vi "Vision Global.vi"() -> ()   [LabVIEW 2018]
uses:
  Vision Data.ctl
panel:
  in  "Track?":bool
  out "Vision Data":T1
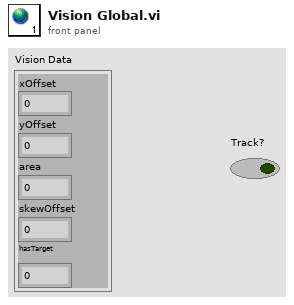
[diagram p1: front panel]
types:
  T1 = typedef "Vision Data.ctl" = cluster{"xOffset":dbl, "yOffset":dbl, "area":dbl, "skewOffset":dbl, "hasTarget":dbl}
diagram:
